vi "Pulse Former.vi"(5 "Input":bool) -> (2 "Pulse":bool)   [LabVIEW 2014]
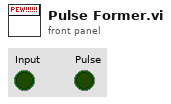
[diagram p1: front panel]
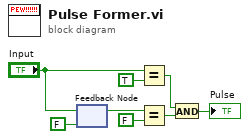
[diagram p0: block diagram]
diagram:
  n1 = feedback-in #1("Input") -> ()
  n2 = feedback #1(FALSE ("Input")) -> (w6:bool)
  n3 = Equal?(x="Input", y=TRUE) -> (x = y?=w3:bool)
  n4 = Equal?(x=w6, y=FALSE) -> (x = y?=w4:bool)
  n5 = And(x=w3, y=w4) -> (x .and. y?=→"Pulse":bool)
